vi "Play Function Block.vi"() -> ()   [LabVIEW 2018]
uses:
  TwinCAT ADS Class/TwinCAT ADS.lvclass
panel:
  out "Value":variant
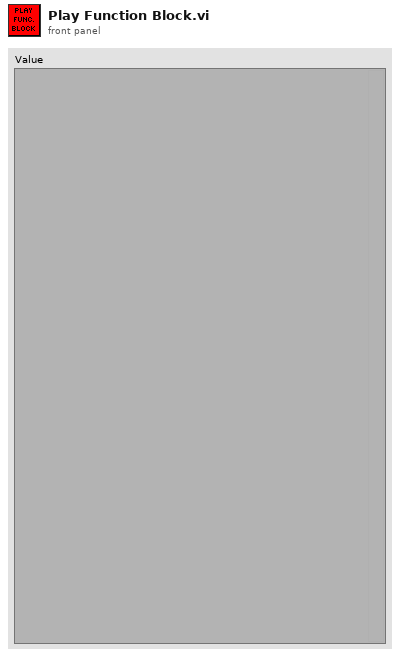
[diagram p1: front panel]
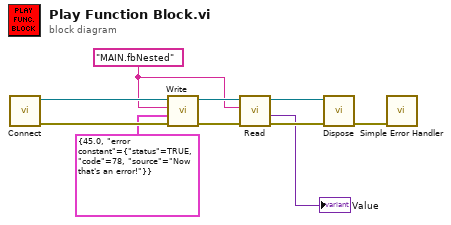
[diagram p0: block diagram]
diagram:
  w1 = "MAIN.fbNested" ("Symbol Name")
  n1 = call "Connect.vi"() -> ("error out"=w7:errorcluster, "TwinCAT ADS out"=w9:refnum<class "TwinCAT ADS.lvclass">)  [unwired: 10 in]
  n2 = call "Write.vi"("error in (no error)"=w7, "Value"=cluster{dbl, "error constant":errorcluster} {45.0, "error constant"={"status"=TRUE, "code"=78, "source"="Now that's an error!"}}, "Symbol Name"=w1, "TwinCAT ADS in"=w9) -> ("error out"=w3:errorcluster, "TwinCAT ADS out"=w4:refnum<class "TwinCAT ADS.lvclass">)  [unwired: 6 in]
  n3 = call "Read.vi"("error in (no error)"=w3, "Symbol Name"=w1, "TwinCAT ADS in"=w4) -> ("error out"=w10:errorcluster, "Value"=→"Value":variant, "TwinCAT ADS out"=w2:refnum<class "TwinCAT ADS.lvclass">)  [unwired: 6 in]
  n4 = call "Dispose.vi"("error in (no error)"=w10, "TwinCAT ADS in"=w2) -> ("error out"=w5:errorcluster)  [unwired: 9 in]
  n5 = call <vilib>:"Simple Error Handler.vi"("error in (no error)"=w5) -> ()  [unwired: 4 in, 5 out]
